vi "WSVCAP SHL Host LL I2C Read.vi"(0 "Bytes to Read":u8=8, 1 "Wait Ticks":u32, 2 "Slave Address":u8, 5 "Sub Address [U8]":u8=191 format="%.0x", 7 "Socket Mask [U64]":u64=1 format="%012x", 11 "error in":errorcluster) -> (4 "C1:1-16 Read Data [DUT Ordered]":u8[][](array[numeric]), 6 "C2:1-16 Read Data [DUT Ordered]":u8[][](array[numeric]), 8 "C3:1-16 Read Data [DUT Ordered]":u8[][](array[numeric]), 10 "Status":u8[](array[numeric]) format="%.0x", 15 "error out":errorcluster)   [LabVIEW 2012]
uses:
  Type Defs/WSVCAP SHL Top Level Write Read State Enum.ctl
  Type Defs/WSVCAP SHL State.ctl
  Type Defs/WSVCAP SHL Transaction Enum.ctl
  Type Defs/WSVCAP SHL Top Level Control Enum.ctl
panel:
  out "Bit Array":u64[](array[numeric]) format="%.0x"
  out "Data Headers":u8[](array[numeric])=[1, 2, 3, 4, 5, 6, 7, 8, 9, 10, 11, 12, 12, 14, 15, 16]
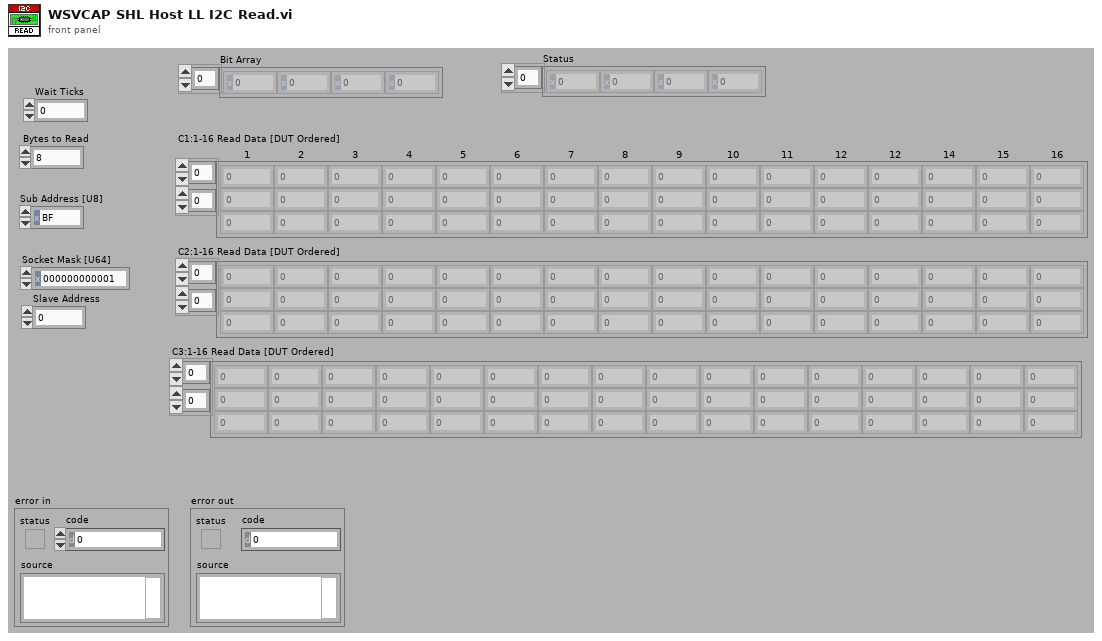
[diagram p1: front panel]
types:
  T1 = typedef "WSVCAP SHL Top Level Write Read State Enum.ctl" = enum16{"Start", "Write", "Read", "Get Status", "Wait Until Done"}
  T2 = typedef "WSVCAP SHL Transaction Enum.ctl" = enum16{"I2C-Read Data", "I2C-Write Data", "SPI-Write/Read Data", "RFFE-Ext Write", "RFFE-Ext Read"}
  T3 = typedef "WSVCAP SHL Top Level Control Enum.ctl" = enum16{"Start", "Cmd", "Transaction", "Wait Ticks", "Socket Mask", "Slave Address", "Sub Address", "Bytes to Write", "Bytes to Read", "Write Data", "Write Flag", "Read Data", "Read Flag", "Ack Read", "Read Status Flag", "Ack Read Status", "Status", "Cycle Count", "Stop Cycle", "Exit"}
  T4 = typedef "WSVCAP SHL State.ctl" = enum8{"Idle", "Transfer Data"}
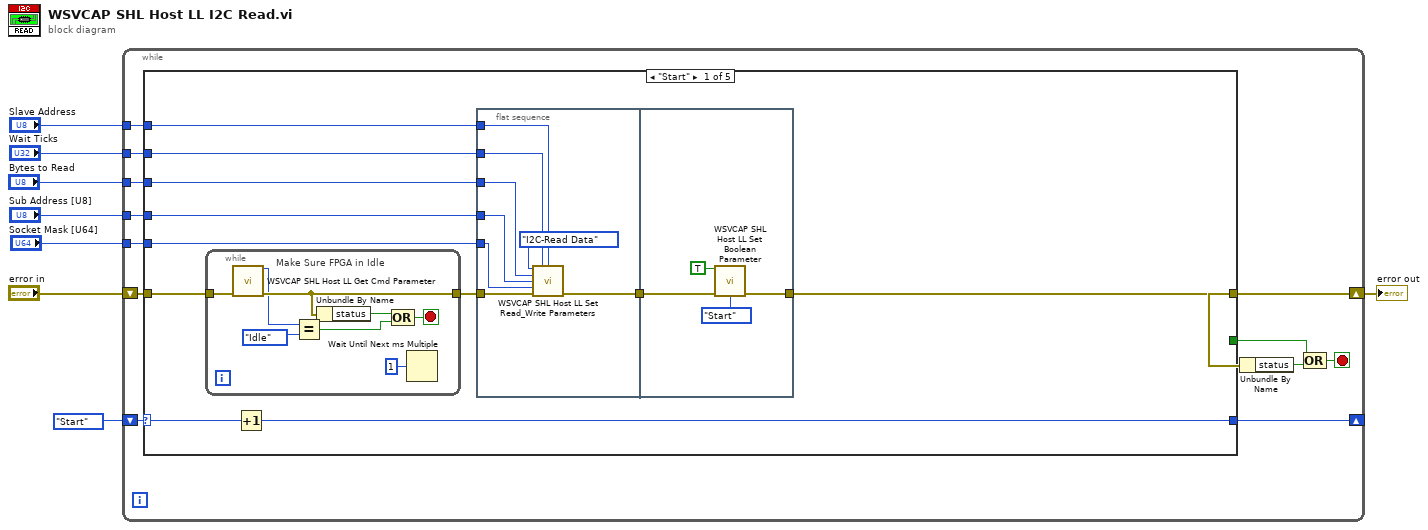
[diagram p0: block diagram]
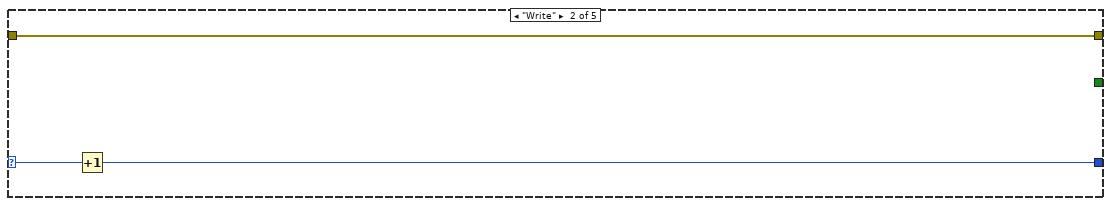
[diagram p2: hidden frame]
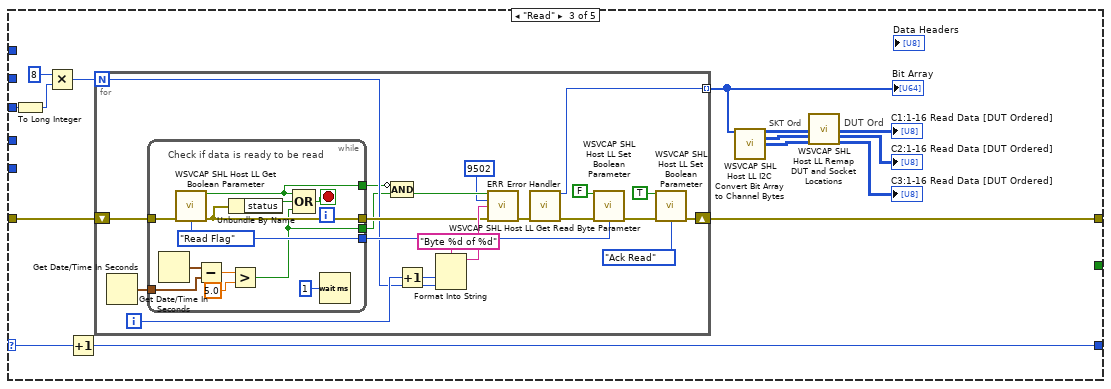
[diagram p3: hidden frame]
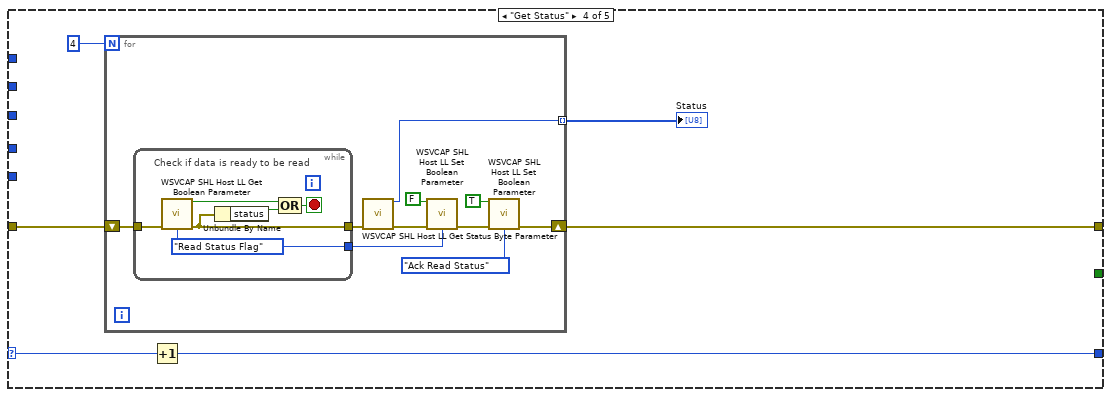
[diagram p4: hidden frame]
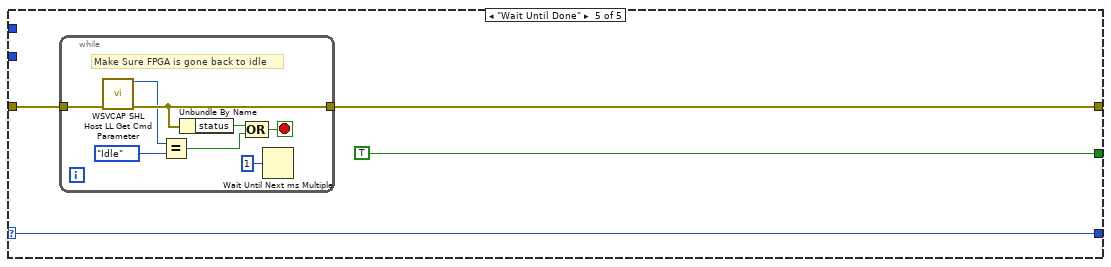
[diagram p5: hidden frame]
diagram:
  n1 = while {
    shift-right: [w19] -> w7
    shift-left: "error in" -> [w20]
    shift-right: [w14] -> _
    shift-left: WSVCAP_SHL_Top_Level_Write_Read_State_Enum."Start" ("Write Read State") -> [w15]
    tunnel: "Bytes to Read" -> [w13]
    tunnel: "Sub Address [U8]" -> [w12]
    tunnel: "Socket Mask [U64]" -> [w11]
    tunnel: "Wait Ticks" -> [w10]
    tunnel: "Slave Address" -> [w9]
    stop <- w16 stop-if-true
    n2 = case shown="\"Start\"" w15 {
      selector: w15 -> [w30 w52 w67 w105 w125]
      tunnel: w20 -> [w31 w51 w56 w107 w127]
      tunnel: [w26 w51 w68 w106 w126] -> w19
      tunnel: [_ _ _ _ TRUE] -> w18
      tunnel: [w29 w53 w66 w104 w125] -> w14
      tunnel: w13 -> [w28 _ w65 _ _]
      tunnel: w12 -> [w24 _ _ _ _]
      tunnel: w11 -> [w23 _ _ _ _]
      tunnel: w10 -> [w22 _ _ _ _]
      tunnel: w9 -> [w21 _ _ _ _]
      frame "Start" {
        n3 = while {
          tunnel: w31 -> [w46]
          tunnel: [w45] -> w27
          stop <- w50 stop-if-true
          # "Make Sure FPGA in Idle"
          n4 = call "WSVCAP SHL Host LL Get Cmd Parameter.vi"("error in (no error)"=w46) -> ("I2C_Cmd"=w44:T4, "error out"=w45:errorcluster)  [unwired: 13 in]
          n5 = Equal?(x=w44, y=WSVCAP_SHL_State."Idle" ("Type")) -> (x = y?=w48:bool)
          n6 = Unbundle By Name(w45) -> ("status"=w43:bool)
          n7 = Compound Arithmetic op=OR(w43, w48) -> (w50:bool)
          n8 = Wait Until Next ms Multiple(millisecond multiple=u32 1) -> ()  [unwired: 1 out]
        }
        n9 = Increment(x=w30) -> (x+1=w29:T1)
        n10 = flat-sequence {
          tunnel: w28 -> [w36]
          tunnel: w27 -> [w39]
          tunnel: [w37] -> w25
          tunnel: w24 -> [w34]
          tunnel: w23 -> [w35]
          tunnel: w22 -> [w33]
          tunnel: w21 -> [w32]
          tunnel: [w42] -> w26
          tunnel: w25 -> [w42]
          frame #0 {
            n11 = call "WSVCAP SHL Host LL Set Read_Write Parameters.vi"("Transaction"=WSVCAP_SHL_Transaction_Enum."I2C-Read Data", "Wait Ticks"=w33, "Slave Address"=w32, "Bytes"=w36, "Sub Address [U8]"=w34, "Socket Mask [U64]"=w35, "error in (no error)"=w39) -> ("error out"=w37:errorcluster)  [unwired: 8 in]
          }
          frame #1 {
            n12 = call "WSVCAP SHL Host LL Set Boolean Parameter.vi"("Boolean In"=TRUE, "error in (no error)"=w42, "FPGA Top Level Control"=WSVCAP_SHL_Top_Level_Control_Enum."Start") -> ()  [unwired: 12 in, 1 out]
          }
        }
      }
      frame "Write" {
        n13 = Increment(x=w52) -> (x+1=w53:T1)
      }
      frame "Read" {
        # "SKT Ord"
        # "DUT Ord"
        n14 = To Long Integer(number=w65) -> (32bit integer=w64:i32)
        n15 = Multiply(x=8, y=w64) -> (x*y=w62:i32)
        n16 = Increment(x=w67) -> (x+1=w66:T1)
        n17 = for {
          N: w62 -> [w72]
          shift-right: [w87] -> w68
          shift-left: w56 -> [w89]
          tunnel: [w81] -> w63 mode=indexing
          i -> [w73]
          n18 = Get Date/Time In Seconds() -> (seconds since 1Jan1904=w69:timestamp)
          n19 = while {
            tunnel: w89 -> [w100]
            tunnel: [w99] -> w75
            tunnel: [w97] -> w86
            tunnel: w69 -> [w94]
            tunnel: [w91] -> w71
            tunnel: [w90] -> w70
            stop <- w101 stop-if-true
            w97 = WSVCAP_SHL_Top_Level_Control_Enum."Read Flag" ("FPGA Top Level Control")
            # "Check if data is ready to be read"
            n20 = Get Date/Time In Seconds() -> (seconds since 1Jan1904=w95:timestamp)
            n21 = call "WSVCAP SHL Host LL Get Boolean Parameter.vi"("error in (no error)"=w100, "FPGA Top Level Control"=w97) -> ("Boolean Out"=w91:bool, "error out"=w99:errorcluster)  [unwired: 12 in]
            n22 = Subtract(x=w95, y=w94) -> (x-y=w93:dbl)
            n23 = Unbundle By Name(w99) -> ("status"=w98:bool)
            n24 = Greater?(x=w93, y=5.0) -> (0:w90:bool)
            n25 = Compound Arithmetic op=OR(w91, w98, w90) -> (w101:bool)
            n26 = Wait (ms)(milliseconds to wait=u32 1) -> ()  [unwired: 1 out]
          }
          n27 = Compound Arithmetic op=AND(invert w71, w70) -> (w80:bool)
          n28 = Increment(x=w73) -> (x+1=w76:i32)
          n29 = Format Into String(format string="Byte %d of %d", w76, w72) -> (resulting string=w78:string)  [unwired: 2 in, 1 out]
          n30 = call "ERR Error Handler.vi"("Error Status"=w80, "Error Code"=9502, "Cause Of Error"=w78, "Error In (no error)"=w75) -> ("Error Out"=w74:errorcluster)  [unwired: 11 in]
          n31 = call "WSVCAP SHL Host LL Get Read Byte Parameter.vi"("error in (no error)"=w74) -> ("Read Data In"=w81:u64, "error out"=w88:errorcluster)  [unwired: 13 in]
          n32 = call "WSVCAP SHL Host LL Set Boolean Parameter.vi"("Boolean In"=FALSE ("Read Flag"), "error in (no error)"=w88, "FPGA Top Level Control"=w86) -> ("error out"=w82:errorcluster)  [unwired: 12 in]
          n33 = call "WSVCAP SHL Host LL Set Boolean Parameter.vi"("Boolean In"=TRUE ("Write Flag"), "error in (no error)"=w82, "FPGA Top Level Control"=WSVCAP_SHL_Top_Level_Control_Enum."Ack Read") -> ("error out"=w87:errorcluster)  [unwired: 12 in]
        }
        "Bit Array" <- w63
        n34 = call "WSVCAP SHL Host LL I2C Convert Bit Array to Channel Bytes.vi"("Bit Array"=w63) -> ("C1:1-16 Read Data [SKT Ordered]"=w60:u8[][], "C2:1-16 Read Data [SKT Ordered]"=w59:u8[][], "C3:1-16 Read Data [SKT Ordered]"=w55:u8[][])  [unwired: 12 in]
        n35 = call "WSVCAP SHL Host LL Remap DUT and Socket Locations.vi"("C1 Socket Ordered Data In"=w60, "C2 Socket Ordered Data In"=w59, "C3 Socket Ordered Data In"=w55) -> ("C1 DUT Ordered Data Out"=→"C1:1-16 Read Data [DUT Ordered]":u8[][], "C2 DUT Ordered Data Out"=→"C2:1-16 Read Data [DUT Ordered]":u8[][], "C3 DUT Ordered Data Out"=→"C3:1-16 Read Data [DUT Ordered]":u8[][])  [unwired: 11 in, 3 out]
      }
      frame "Get Status" {
        n36 = for {
          N: 4 -> [_]
          shift-right: [w114] -> w106
          shift-left: w107 -> [w117]
          tunnel: [w108] -> w103 mode=indexing
          n37 = while {
            tunnel: w117 -> [w121]
            tunnel: [w120] -> w116
            tunnel: [w118] -> w113
            stop <- w123 stop-if-true
            w118 = WSVCAP_SHL_Top_Level_Control_Enum."Read Status Flag" ("FPGA Top Level Control")
            # "Check if data is ready to be read"
            n38 = call "WSVCAP SHL Host LL Get Boolean Parameter.vi"("error in (no error)"=w121, "FPGA Top Level Control"=w118) -> ("Boolean Out"=w122:bool, "error out"=w120:errorcluster)  [unwired: 12 in]
            n39 = Unbundle By Name(w120) -> ("status"=w119:bool)
            n40 = Compound Arithmetic op=OR(w122, w119) -> (w123:bool)
          }
          n41 = call "WSVCAP SHL Host LL Get Status Byte Parameter.vi"("error in (no error)"=w116) -> ("I2C Status Byte"=w108:u8, "error out"=w115:errorcluster)  [unwired: 13 in]
          n42 = call "WSVCAP SHL Host LL Set Boolean Parameter.vi"("Boolean In"=FALSE ("Read Flag"), "error in (no error)"=w115, "FPGA Top Level Control"=w113) -> ("error out"=w109:errorcluster)  [unwired: 12 in]
          n43 = call "WSVCAP SHL Host LL Set Boolean Parameter.vi"("Boolean In"=TRUE ("Write Flag"), "error in (no error)"=w109, "FPGA Top Level Control"=WSVCAP_SHL_Top_Level_Control_Enum."Ack Read Status") -> ("error out"=w114:errorcluster)  [unwired: 12 in]
        }
        "Status" <- w103
        n44 = Increment(x=w105) -> (x+1=w104:T1)
      }
      frame "Wait Until Done" {
        n45 = while {
          tunnel: w127 -> [w130]
          tunnel: [w129] -> w126
          stop <- w132 stop-if-true
          # "Make Sure FPGA is gone back to idle"
          n46 = call "WSVCAP SHL Host LL Get Cmd Parameter.vi"("error in (no error)"=w130) -> ("I2C_Cmd"=w128:T4, "error out"=w129:errorcluster)  [unwired: 13 in]
          n47 = Equal?(x=w128, y=WSVCAP_SHL_State."Idle") -> (x = y?=w133:bool)
          n48 = Unbundle By Name(w129) -> ("status"=w134:bool)
          n49 = Compound Arithmetic op=OR(w134, w133) -> (w132:bool)
          n50 = Wait Until Next ms Multiple(millisecond multiple=u32 1) -> ()  [unwired: 1 out]
        }
      }
    }
    n51 = Unbundle By Name(w19) -> ("status"=w17:bool)
    n52 = Compound Arithmetic op=OR(w18, w17) -> (w16:bool)
  }
  "error out" <- w7
